vi "NI VeriStand - Search for All Items by GUID.vi"(8 "error in":errorcluster, 9 "Find All? (T)":bool=TRUE, 10 "Item GUID":string, 11 "Section Ref in":T1 format="%.0x") -> (0 "error out":errorcluster, 2 "Item Refs":T1[](array[typedef]) format="%.0x", 3 "Section Ref out":T1 format="%.0x", 4 "Found":bool)   [LabVIEW 2020, in "Custom Device Utility Library.lvlib"]
doc: "Searches a custom device section for the item(s) you specify. You can search for one or multiple items by name, GUID, or property name and value. You must manually select the polymorphic instance to use."
uses:
  <vilib>/NI VeriStand/Custom Device Tools/Custom Device Utility Library/Custom Device Utility Library.lvlib
  <vilib>/NI VeriStand/Custom Device API/Custom Device Item Ref.ctl
  <vilib>/NI VeriStand/Custom Device API/Custom Device API.lvlib
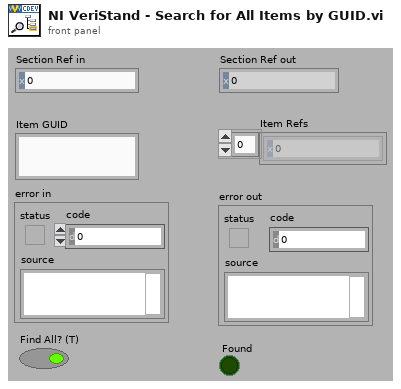
[diagram p1: front panel]
types:
  T1 = typedef "Custom Device API.lvlib/Custom Device Item Ref.ctl" = u64
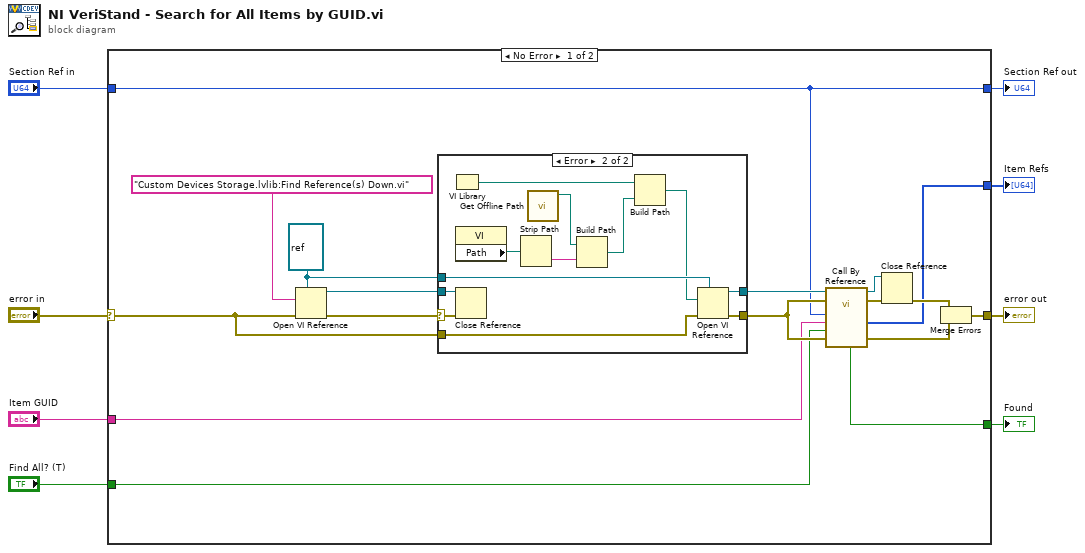
[diagram p0: block diagram]
diagram:
  n1 = case shown="No Error" "error in" {
    selector: "error in" -> [w15 w41]
    tunnel: [w20 w41] -> w8
    tunnel: "Section Ref in" -> [w14 w40]
    tunnel: [w19 _] -> w6
    tunnel: "Item GUID" -> [w18 _]
    tunnel: [w17 _] -> w4
    tunnel: "Find All? (T)" -> [w16 _]
    tunnel: [w14 w40] -> w1
    frame No Error {
      w10 = refnum<vi> refnum ("type specifier VI Refnum (for type only)")
      n2 = Open VI Reference(type specifier VI Refnum (for type only)=w10, vi path="Custom Devices Storage.lvlib:Find Reference(s) Down.vi", error in (no error)=w15) -> (vi reference=w11:refnum<vi>, error out=w12:errorcluster)  [unwired: 3 out]
      n3 = case shown="Error" w12 {
        selector: w12 -> [w26 w36]
        tunnel: w10 -> [_ w38]
        tunnel: w11 -> [w27 w37]
        tunnel: [w27 w35] -> w22
        tunnel: [w26 w34] -> w23
        tunnel: w15 -> [_ w39]
        frame No Error {
        }
        frame Error {
          n4 = VI Library() -> (path=w33:path)
          n5 = property class="VI"() -> ("Path"=w30:path)  [unwired: 2 in, 2 out]
          n6 = Close Reference(reference=w37, error in (no error)=w36) -> ()  [unwired: 1 out]
          n7 = Strip Path(path=w30) -> (name=w29:string)  [unwired: 1 out]
          n8 = call <vilib>:"Get Offline Path.vi"() -> ("Offline Path"=w28:path)  [unwired: 11 in]
          n9 = Build Path(base path=w28, name or relative path=w29) -> (appended path=w32:path)
          n10 = Build Path(base path=w33, name or relative path=w32) -> (appended path=w31:path)
          n11 = Open VI Reference(type specifier VI Refnum (for type only)=w38, vi path=w31, error in (no error)=w39) -> (vi reference=w35:refnum<vi>, error out=w34:errorcluster)  [unwired: 3 out]
        }
      }
      n12 = call-by-ref "?"(reference=w22, error in=w23, 8:"error in (no error)"=w23, "Find All?"=w16, "Item GUID"=w18, "Section Ref in"=w14) -> (reference out=w9:refnum<vi>, error out=w24:errorcluster, 0:"error out"=w21:errorcluster, "Item Refs"=w17:T1[], "Found"=w19:bool)  [unwired: 4 in, 1 out]
      n13 = Close Reference(reference=w9, error in (no error)=w24) -> (error out=w25:errorcluster)
      n14 = Merge Errors(w25, w21) -> (w20:errorcluster)
    }
    frame Error {
    }
  }
  "Found" <- w6
  "error out" <- w8
  "Section Ref out" <- w1
  "Item Refs" <- w4
